vi "LVClass_Camera get TriggerMode.vi"(0 "Camera in":refnum<class "Camera.lvclass">, 11 "error in (no error)":errorcluster) -> (4 "Camera out":refnum<class "Camera.lvclass">, 8 "Trigger Mode":string, 15 "error out":errorcluster)   [LabVIEW 2020, in "Camera.lvclass"]
doc: "Get camera trigger mode\n\n<B>CameraIn</B> : Camera object.\n<B>CameraOut</B> : Camera object.\n<B>Trigger Mode</B> : trigger mode value (Internal, Rising edge, Falling edge, Software, High level, Low level)"
uses:
  Camera.lvclass
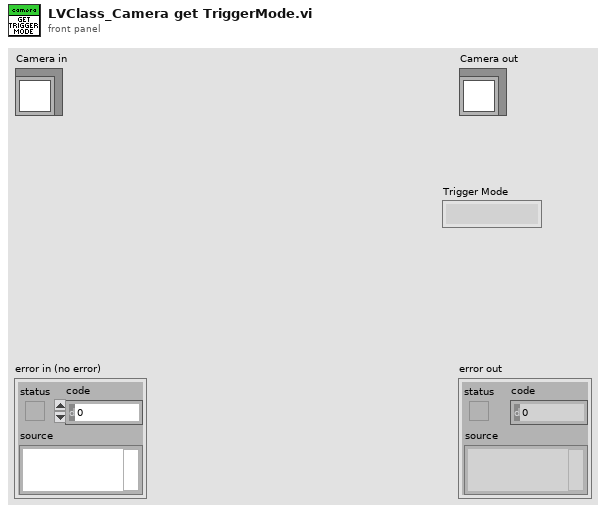
[diagram p1: front panel]
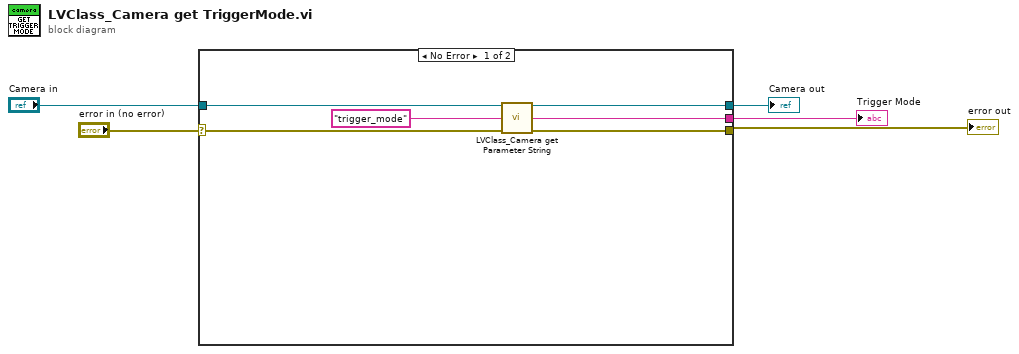
[diagram p0: block diagram]
diagram:
  n1 = case shown="No Error" "error in (no error)" {
    selector: "error in (no error)" -> [w8 w13]
    tunnel: [w7 w13] -> w4
    tunnel: [w10 w12] -> w2
    tunnel: "Camera in" -> [w11 w12]
    tunnel: [w6 _] -> w1
    frame No Error {
      n2 = call "LVClass_Camera get Parameter String.vi"("Camera in"=w11, "parameter_name"="trigger_mode", "error in (no error)"=w8) -> ("Camera out"=w10:refnum<class "Camera.lvclass">, "value"=w6:string, "error out"=w7:errorcluster)  [unwired: 10 in]
    }
    frame Error {
    }
  }
  "error out" <- w4
  "Camera out" <- w2
  "Trigger Mode" <- w1
